vi "Update Error Message Icon.vi"(8 "error in (no error)":errorcluster, 10 "selected row":i32, 11 "statusListbox in":refnum<vi>) -> (0 "error out":errorcluster, 3 "open?":bool)   [LabVIEW 2021, in "MeasurementClient Editor.lvlib"]
uses:
  MeasurementClient Editor.lvlib
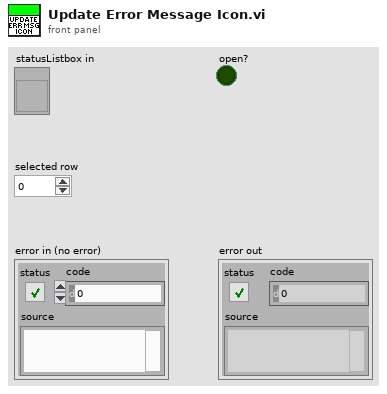
[diagram p1: front panel]
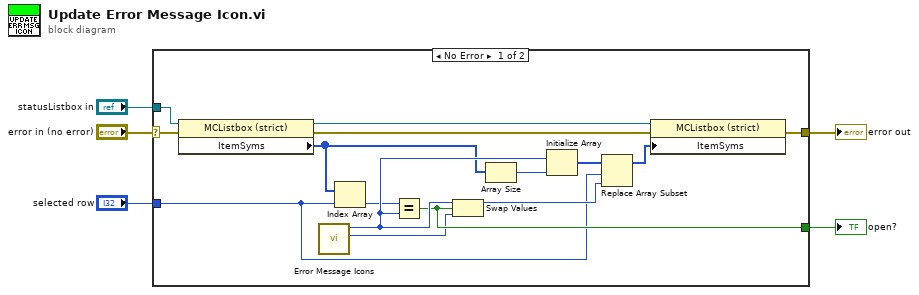
[diagram p0: block diagram]
diagram:
  n1 = case shown="No Error" "error in (no error)" {
    selector: "error in (no error)" -> [w17 w21]
    tunnel: [w19 _] -> w5
    tunnel: [w18 w21] -> w4
    tunnel: "selected row" -> [w14 _]
    tunnel: "statusListbox in" -> [w8 _]
    frame No Error {
      n2 = property class="MCListbox (strict)"(reference=w8, error in=w17) -> (reference out=w7:refnum<vi>, error out=w6:errorcluster, "ItemSyms"=w11:i32[])
      n3 = call "Error Message Icons.vi"() -> ("open"=w10:i32, "closed"=w20:i32)  [unwired: 10 in]
      n4 = Index Array(array=w11, index=w14) -> (element=w9:i32)
      n5 = Equal?(x=w9, y=w20) -> (x = y?=w19:bool)
      n6 = Swap Values(12:w20, 13:w19, 14:w10) -> (1:w15:i32)  [unwired: 1 out]
      n7 = Array Size(array=w11) -> (size(s)=w12:i32)
      n8 = Initialize Array(w20, w12) -> (w13:i32[])
      n9 = Replace Array Subset(array=w13, new element=w15, index=w14) -> (w16:i32[])
      n10 = property class="MCListbox (strict)"(reference=w7, error in=w6, "ItemSyms"=w16) -> (error out=w18:errorcluster)  [unwired: 1 out]
    }
    frame Error {
    }
  }
  "open?" <- w5
  "error out" <- w4
